vi "StartCAN.1.vi"(11 "CAN Interface":refnum<k21>="CAN1") -> (0 "error out":errorcluster, 1 "Tester Write Session out":refnum<k21>, 2 "Read Session out":refnum<k21>, 3 "DSC Write Session out":refnum<k21>)   [LabVIEW 2018]
uses:
  <vilib>/xnet/xnet.llb/XNET CAN Comm State.ctl
  <vilib>/xnet/xnet.llb/XNET Control Scope.ctl
  <vilib>/xnet/xnet.llb/XNET Frame CAN.ctl
  <vilib>/xnet/xnet.llb/XNET Frame Type CAN.ctl
  <vilib>/xnet/xnet.llb/XNET Create Session (Frame Input Queued).vi
  <vilib>/xnet/xnet.llb/XNET Create Session (Frame Output Single-point).vi
  <vilib>/xnet/xnet.llb/XNET Write (Frame CAN).vi
  <vilib>/xnet/xnet.llb/XNET Read (State CAN Comm).vi
  <vilib>/xnet/xnet.llb/XNET Wait (Interface Communicating).vi
  <resource>/objmgr/xnet.rc
panel:
  in  "error in (no error)":errorcluster
  out "TesterPresentSession":refnum<k21>
  out "CAN:I/O Mode":u32(ring) items=["CAN 2.0", "CAN FD", "CAN FD+BRS"]
  out "Protocol":u32(ring) items=["CAN", "FlexRay", "LIN"]
  out "CAN:Transceiver Capability":u32(ring) items=["HS"=0, "LS"=1, "XS"=3, "XS (HS/LS)"=4]
  out "Interface:CAN:Transceiver State":u32(ring) items=["Normal", "Sleep", "Single Wire Wakeup", "Single Wire High-Speed"]
  out "Interface:CAN:Transceiver State 2":u32(ring) items=["Normal", "Sleep", "Single Wire Wakeup", "Single Wire High-Speed"]
  out "Interface:CAN:Transceiver State 3":u32(ring) items=["Normal", "Sleep", "Single Wire Wakeup", "Single Wire High-Speed"]
  out "CAN:Termination Capability":u32(ring) items=["No", "Yes"]
  out "Array":T1[](array[typedef]) items=["Error Active", "Error Passive", "Bus Off", "Init"]
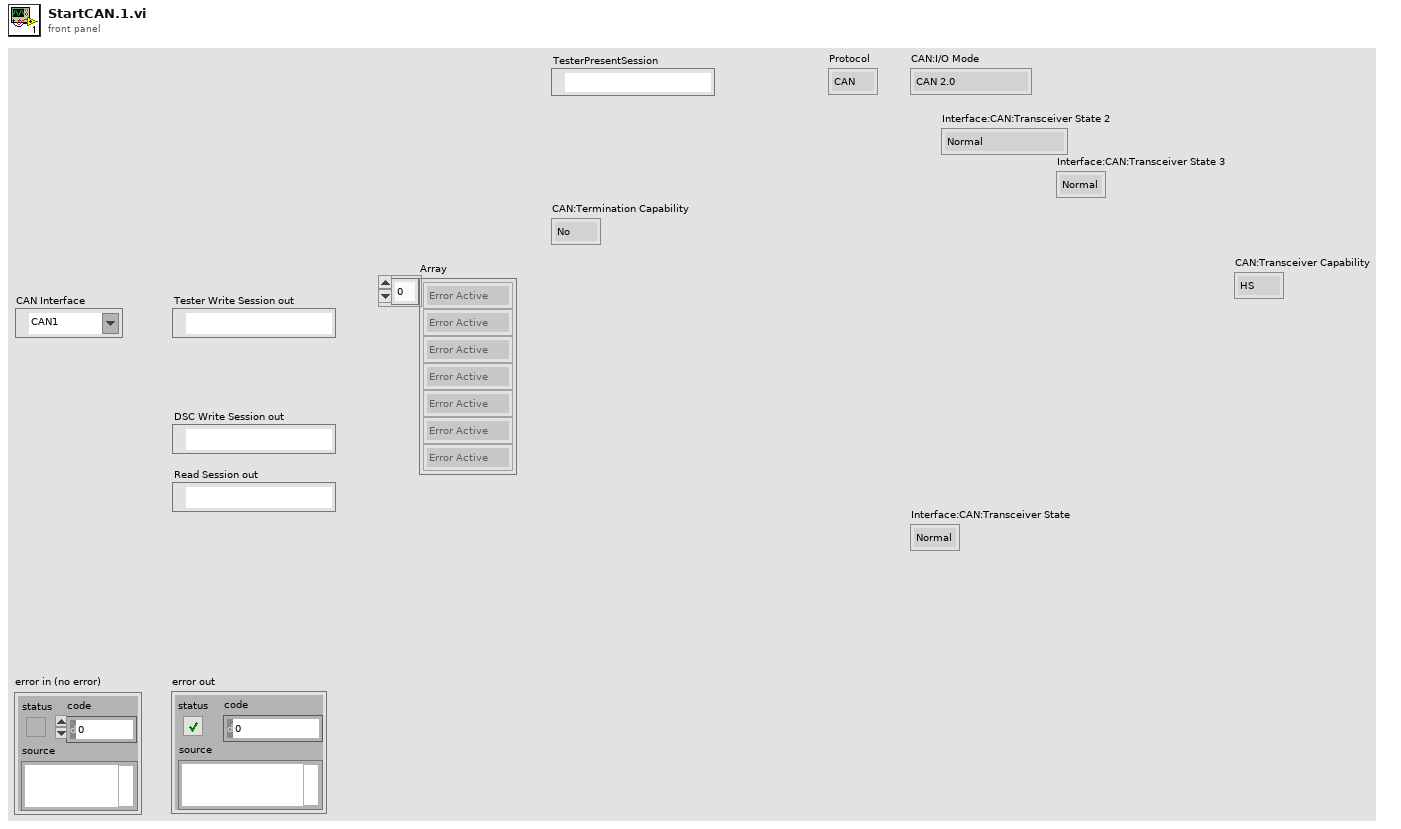
[diagram p1: front panel]
types:
  T1 = typedef "XNET CAN Comm State.ctl" = u8
  T2 = typedef "XNET Frame CAN.ctl" = cluster{"timestamp":timestamp, "payload":u8[], "identifier":u32, "type":T3, "extended?":bool, "echo?":bool}
  T3 = typedef "XNET Frame Type CAN.ctl" = u8
  T4 = typedef "XNET Control Scope.ctl" = u32
  T5 = cluster{"Comment":string, "Default Payload":u8[], "Identifier":u32, "Name (Short)":string, "Payload Length":u32, "PDU_Mapping":cluster{"PDU":string, "Start Bit":u32, "Update Bit":i32}[], "CAN:Extended Identifier?":bool, "CAN:Timing Type":u32, "CAN:Transmit Time":dbl, "CAN:I/O Mode":u32}
  T6 = typedef "XNET CAN Comm.ctl" = cluster{"fault code":i32, "fault?":bool, "communication state":T1, "last error":T7, "receive error counter":u8, "transmit error counter":u8, "transceiver error?":bool, "sleep?":bool}
  T7 = typedef "XNET CAN Last Err.ctl" = u8
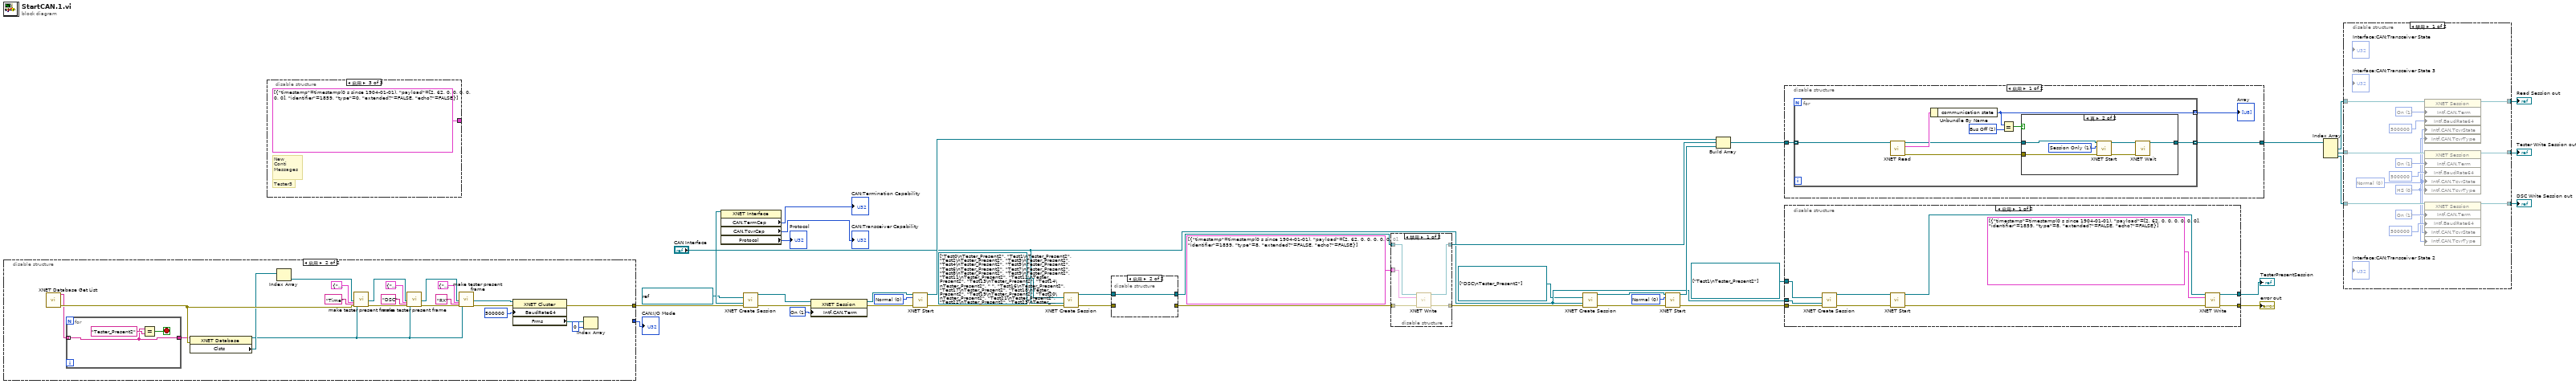
[diagram p0: block diagram]
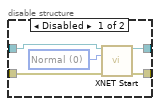
[diagram p3: hidden frame]
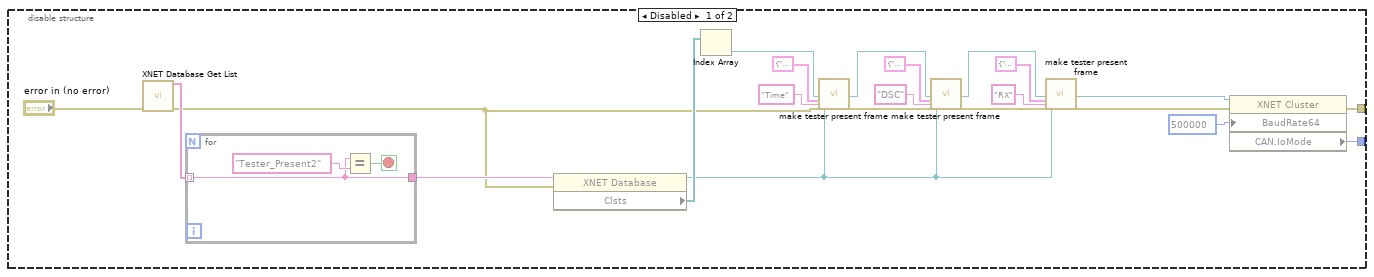
[diagram p4: hidden frame]
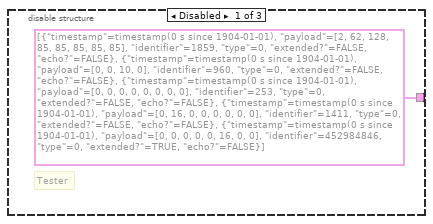
[diagram p9: hidden frame]
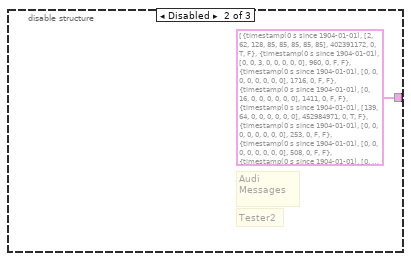
[diagram p10: hidden frame]
diagram:
  w11 = u32 1 items=["Off", "On"] ("Interface:CAN:Termination")
  w29 = T4 0 items=["Normal", "Session Only", "Interface Only", "Session Only Blocking"] ("scope (normal)")
  w30 = T4 0 items=["Normal", "Session Only", "Interface Only", "Session Only Blocking"] ("scope (normal)")
  n1 = disable-structure shown="启用" {
    disable-tunnel: [w60 w66] -> w40
    disable-tunnel: [w41 _] -> w15
    frame Disabled {
      n2 = call <vilib>:"XNET Database Get List.vi"("error in (no error)"="error in (no error)") -> ("array of alias"=w50:string[], "error out"=w46:errorcluster)  [unwired: 12 in, 1 out]
      n3 = for {
        tunnel: w50 -> [w63] mode=indexing
        tunnel: [w63] -> w49
        stop <- w64 stop-if-true
        n4 = Equal?(x=w63, y="Tester_Present2") -> (x = y?=w64:bool)
      }
      n5 = property class="XNET Database"(reference=w49, error in=w46) -> (reference out=w42:refnum<k21>, "Clsts"=w61:refnum<k21>[])  [unwired: 1 out]
      n6 = Index Array(array=w61) -> (element=w44:refnum<k21>)  [unwired: 1 in]
      n7 = call <userlib>:"make tester present frame.vi"("Cluster::"=w44, "New Frame Properties"=T5 {"Comment"="DSC", "Default Payload"=[0, 0, 0, 0, 0, 0, 0, 0], "Identifier"=1714, "Name (Short)"="Time", "Payload Length"=8, "PDU_Mapping"=[], "CAN:Extended Identifier?"=FALSE, "CAN:Timing Type"=0, "CAN:Transmit Time"=0.001, "CAN:I/O Mode"=0}, "frame name"="Time", "error in (no error)"=w46, "database in"=w42) -> ("target cluster out"=w43:refnum<k21>, "error out"=w45:errorcluster)  [unwired: 21 in]
      n8 = call <userlib>:"make tester present frame.vi"("Cluster::"=w43, "New Frame Properties"=T5 {"Comment"="DSC", "Default Payload"=[0, 0, 0, 0, 0, 0, 0, 0], "Identifier"=402391172, "Name (Short)"="DSC", "Payload Length"=8, "PDU_Mapping"=[], "CAN:Extended Identifier?"=TRUE, "CAN:Timing Type"=1, "CAN:Transmit Time"=0.001, "CAN:I/O Mode"=0}, "frame name"="DSC", "error in (no error)"=w45, "database in"=w42) -> ("target cluster out"=w59:refnum<k21>, "error out"=w58:errorcluster)  [unwired: 21 in]
      n9 = call <userlib>:"make tester present frame.vi"("Cluster::"=w59, "New Frame Properties"=T5 {"Comment"="RX", "Default Payload"=[0, 127, 0, 0, 0, 0, 0, 0], "Identifier"=402522244, "Name (Short)"="RX", "Payload Length"=8, "PDU_Mapping"=[], "CAN:Extended Identifier?"=TRUE, "CAN:Timing Type"=1, "CAN:Transmit Time"=0.001, "CAN:I/O Mode"=0}, "frame name"="RX", "error in (no error)"=w58, "database in"=w42) -> ("target cluster out"=w52:refnum<k21>, "error out"=w51:errorcluster)  [unwired: 21 in]
      n10 = property class="XNET Cluster"(reference=w52, error in=w51, "BaudRate64"=u64 500000 ("64bit Baud Rate")) -> (error out=w60:errorcluster, "CAN.IoMode"=w41:u32)  [unwired: 1 out]
    }
    frame Enabled {
      n11 = call <vilib>:"XNET Database Get List.vi"() -> ("array of alias"=w84:string[], "error out"=w85:errorcluster)  [unwired: 13 in, 1 out]
      n12 = for {
        tunnel: w84 -> [w88] mode=indexing
        tunnel: [w88] -> w71
        stop <- w89 stop-if-true
        n13 = Equal?(x=w88, y="Tester_Present2") -> (x = y?=w89:bool)
      }
      n14 = property class="XNET Database"(reference=w71, error in=w85) -> (reference out=w68:refnum<k21>, "Clsts"=w72:refnum<k21>[])  [unwired: 1 out]
      n15 = Index Array(array=w72) -> (element=w87:refnum<k21>)  [unwired: 1 in]
      n16 = call <userlib>:"make tester present frame.vi"("Cluster::"=w87, "New Frame Properties"=T5 {"Comment"="Time", "Default Payload"=[0, 0, 0, 0, 0, 0, 0, 0], "Identifier"=1859, "Name (Short)"="Time", "Payload Length"=8, "PDU_Mapping"=[], "CAN:Extended Identifier?"=FALSE, "CAN:Timing Type"=0, "CAN:Transmit Time"=0.1, "CAN:I/O Mode"=0}, "frame name"="Time", "error in (no error)"=w85, "database in"=w68) -> ("target cluster out"=w67:refnum<k21>, "error out"=w86:errorcluster)  [unwired: 21 in]
      n17 = call <userlib>:"make tester present frame.vi"("Cluster::"=w67, "New Frame Properties"=T5 {"Comment"="DSC", "Default Payload"=[0, 0, 0, 16, 1, 0, 0, 0], "Identifier"=1859, "Name (Short)"="DSC", "Payload Length"=8, "PDU_Mapping"=[], "CAN:Extended Identifier?"=FALSE, "CAN:Timing Type"=1, "CAN:Transmit Time"=0.001, "CAN:I/O Mode"=0}, "frame name"="DSC", "error in (no error)"=w86, "database in"=w68) -> ("target cluster out"=w80:refnum<k21>, "error out"=w81:errorcluster)  [unwired: 21 in]
      n18 = call <userlib>:"make tester present frame.vi"("Cluster::"=w80, "New Frame Properties"=T5 {"Comment"="RX", "Default Payload"=[0, 127, 0, 0, 0, 0, 0, 0], "Identifier"=1867, "Name (Short)"="RX", "Payload Length"=8, "PDU_Mapping"=[], "CAN:Extended Identifier?"=FALSE, "CAN:Timing Type"=1, "CAN:Transmit Time"=0.001, "CAN:I/O Mode"=0}, "frame name"="RX", "error in (no error)"=w81, "database in"=w68) -> ("target cluster out"=w82:refnum<k21>, "error out"=w83:errorcluster)  [unwired: 21 in]
      n19 = property class="XNET Cluster"(reference=w82, error in=w83, "BaudRate64"=u64 500000 ("64bit Baud Rate")) -> (error out=w66:errorcluster, "Frms"=w70:refnum<k21>[])  [unwired: 1 out]
      n20 = Index Array(array=w70, index=0 ("索引")) -> ()  [unwired: 1 out]
    }
  }
  "CAN:I/O Mode" <- w15
  n21 = disable-structure shown="启用" {
    disable-tunnel: [T2[] [{"timestamp"=timestamp(0 s since 1904-01-01), "payload"=[2, 62, 128, 85, 85, 85, 85, 85], "identifier"=1859, "type"=0, "extended?"=FALSE, "echo?"=FALSE}, {"timestamp"=timestamp(0 s since 1904-01-01), "payload"=[0, 0, 10, 0], "identifier"=960, "type"=0, "extended?"=FALSE, "echo?"=FALSE}, {"timestamp"=timestamp(0 s since 1904-01-01), "payload"=[0, 0, 0, 0, 0, 0, 0, 0], "identifier"=253, "type"=0, "extended?"=FALSE, "echo?"=FALSE}, {"timestamp"=timestamp(0 s since 1904-01-01), "payload"=[0, 16, 0, 0, 0, 0, 0, 0], "identifier"=1411, "type"=0, "extended?"=FALSE, "echo?"=FALSE}, {"timestamp"=timestamp(0 s since 1904-01-01), "payload"=[0, 0, 0, 0, 0, 16, 0, 0], "identifier"=452984846, "type"=0, "extended?"=TRUE, "echo?"=FALSE}] ("data") T2[] [{"timestamp"=timestamp(0 s since 1904-01-01), "payload"=[2, 62, 128, 85, 85, 85, 85, 85], "identifier"=402391172, "type"=0, "extended?"=TRUE, "echo?"=FALSE}, {"timestamp"=timestamp(0 s since 1904-01-01), "payload"=[0, 0, 3, 0, 0, 0, 0, 0], "identifier"=960, "type"=0, "extended?"=FALSE, "echo?"=FALSE}, {"timestamp"=timestamp(0 s since 1904-01-01), "payload"=[0, 0, 0, 0, 0, 0, 0, 0], "identifier"=1716, "type"=0, "extended?"=FALSE, "echo?"=FALSE}, {"timestamp"=timestamp(0 s since 1904-01-01), "payload"=[0, 16, 0, 0, 0, 0, 0, 0], "identifier"=1411, "type"=0, "extended?"=FALSE, "echo?"=FALSE}, {"timestamp"=timestamp(0 s since 1904-01-01), "payload"=[139, 64, 0, 0, 0, 0, 0, 0], "identifier"=452984971, "type"=0, "extended?"=TRUE, "echo?"=FALSE}, {"timestamp"=timestamp(0 s since 1904-01-01), "payload"=[0, 0, 0, 0, 0, 0, 0, 0], "identifier"=253, "type"=0, "extended?"=FALSE, "echo?"=FALSE}, {"timestamp"=timestamp(0 s since 1904-01-01), "payload"=[0, 0, 0, 0, 0, 0, 0, 0], "identifier"=508, "type"=0, "extended?"=FALSE, "echo?"=FALSE}, {"timestamp"=timestamp(0 s since 1904-01-01), "payload"=[0, 0, 0, 0, 150, 0, 0, 0], "identifier"=1646, "type"=0, "extended?"=FALSE, "echo?"=FALSE}, {"timestamp"=timestamp(0 s since 1904-01-01), "payload"=[0, 0, 0, 0, 0, 0, 0, 150], "identifier"=1719, "type"=0, "extended?"=FALSE, "echo?"=FALSE}, {"timestamp"=timestamp(0 s since 1904-01-01), "payload"=[0, 0, 4, 0, 0, 0, 0, 0], "identifier"=958, "type"=0, "extended?"=FALSE, "echo?"=FALSE}, {"timestamp"=timestamp(0 s since 1904-01-01), "payload"=[0, 0, 0, 0, 0, 0, 0, 0], "identifier"=1635, "type"=0, "extended?"=FALSE, "echo?"=FALSE}, {"timestamp"=timestamp(0 s since 1904-01-01), "payload"=[0, 0, 0, 0, 0, 0, 0, 0], "identifier"=319, "type"=0, "extended?"=FALSE, "echo?"=FALSE}, {"timestamp"=timestamp(0 s since 1904-01-01), "payload"=[0, 0, 0, 0, 0, 0, 0, 0], "identifier"=1616, "type"=0, "extended?"=FALSE, "echo?"=FALSE}, {"timestamp"=timestamp(0 s since 1904-01-01), "payload"=[0, 12, 0, 0, 0, 0, 0, 0], "identifier"=1413, "type"=0, "extended?"=FALSE, "echo?"=FALSE}, {"timestamp"=timestamp(0 s since 1904-01-01), "payload"=[0, 0, 0, 0, 0, 0, 0, 0], "identifier"=1462, "type"=0, "extended?"=FALSE, "echo?"=FALSE}, {"timestamp"=timestamp(0 s since 1904-01-01), "payload"=[16, 64, 0, 0, 0, 16, 0, 0], "identifier"=452984848, "type"=0, "extended?"=TRUE, "echo?"=FALSE}, {"timestamp"=timestamp(0 s since 1904-01-01), "payload"=[0, 0, 0, 0, 0, 0, 0, 0], "identifier"=976, "type"=0, "extended?"=FALSE, "echo?"=FALSE}, {"timestamp"=timestamp(0 s since 1904-01-01), "payload"=[0, 0, 0, 0, 0, 0, 0, 0], "identifier"=974, "type"=0, "extended?"=FALSE, "echo?"=FALSE}, {"timestamp"=timestamp(0 s since 1904-01-01), "payload"=[74, 64, 0, 0, 0, 0, 0, 0], "identifier"=452984906, "type"=0, "extended?"=TRUE, "echo?"=FALSE}, {"timestamp"=timestamp(0 s since 1904-01-01), "payload"=[0, 0, 0, 0, 0, 0, 0, 0], "identifier"=977, "type"=0, "extended?"=FALSE, "echo?"=FALSE}, {"timestamp"=timestamp(0 s since 1904-01-01), "payload"=[0, 0, 0, 0, 0, 0, 0, 0], "identifier"=975, "type"=0, "extended?"=FALSE, "echo?"=FALSE}, {"timestamp"=timestamp(0 s since 1904-01-01), "payload"=[75, 64, 0, 0, 0, 0, 0, 0], "identifier"=452984907, "type"=0, "extended?"=TRUE, "echo?"=FALSE}] ("Array 3") T2[] [{"timestamp"=timestamp(0 s since 1904-01-01), "payload"=[2, 62, 0, 0, 0, 0, 0, 0], "identifier"=1859, "type"=0, "extended?"=FALSE, "echo?"=FALSE}] ("data")] -> _
    frame Disabled {
      # "Tester"
    }
    frame Disabled {
      # "Tester2"
      # "Audi\nMessages"
    }
    frame Enabled {
      # "Tester3"
      # "New\nConti\nMessages"
    }
  }
  n22 = property class="XNET Interface"(reference="CAN Interface") -> ("CAN.TermCap"=→"CAN:Termination Capability":u32, "CAN.TcvrCap"=→"CAN:Transceiver Capability":u32, "Protocol"=→"Protocol":u32)  [unwired: 1 in, 2 out]
  n23 = call-poly <vilib>:"XNET Create Session.vi"("frame"=refnum<k21> "RX\nTester_Present2" ("XNET Frame"), "interface"="CAN Interface", "error in (no error)"=w40) -> ("session out"=w14:refnum<k21>, "error out"=w12:errorcluster)  [unwired: 11 in]
  n24 = property class="XNET Session"(reference=w14, error in=w12, "Intf.CAN.Term"=w11) -> (reference out=w13:refnum<k21>, error out=w10:errorcluster)
  n25 = call <vilib>:"XNET Start.vi"("session in"=w13, "scope (normal)"=w30, "error in (no error)"=w10) -> ("session out"=w37:refnum<k21>, "error out"=w32:errorcluster)  [unwired: 11 in]
  n26 = call-poly <vilib>:"XNET Create Session.vi"("frame list"=refnum<k21>[] ["Test0\nTester_Present2", "Test1\nTester_Present2", "Test2\nTester_Present2", "Test3\nTester_Present2", "Test4\nTester_Present2", "Test5\nTester_Present2", "Test6\nTester_Present2", "Test7\nTester_Present2", "Test8\nTester_Present2", "Test9\nTester_Present2", "Test11\nTester_Present2", "Test12\nTester_Present2", "Test13\nTester_Present2", "Test14\nTester_Present2", " ", "Test16\nTester_Present2", "Test17\nTester_Present2", "Test18\nTester_Present2", "Test19\nTester_Present2", "Test20\nTester_Present2", "Test21\nTester_Present2", "Test22\nTester_Present2", "Test23\nTester_Present2", "Test24\nTester_Present2", "Test25\nTester_Present2", "Test26\nTester_Present2", "Test27\nTester_Present2"] ("Frames"), "interface"="CAN Interface", "error in (no error)"=w32) -> ("session out"=w27:refnum<k21>, "error out"=w28:errorcluster)  [unwired: 11 in]
  n27 = disable-structure shown="启用" {
    disable-tunnel: [w98 w99] -> w39
    disable-tunnel: [w97 _] -> w38
    disable-tunnel: w28 -> [w95 _]
    disable-tunnel: w27 -> [w94 w99]
    frame Disabled {
      w96 = T4 0 items=["Normal", "Session Only", "Interface Only", "Session Only Blocking"] ("scope (normal)")
      n28 = call <vilib>:"XNET Start.vi"("session in"=w94, "scope (normal)"=w96, "error in (no error)"=w95) -> ("session out"=w98:refnum<k21>, "error out"=w97:errorcluster)  [unwired: 11 in]
    }
    frame Enabled {
    }
  }
  n29 = disable-structure shown="禁用" {
    disable-tunnel: w39 -> [w104 w105]
    disable-tunnel: w38 -> [w103 w106]
    disable-tunnel: [w102 w105] -> w36
    disable-tunnel: [w101 w106] -> w31
    disable-tunnel: T2[] [{"timestamp"=timestamp(0 s since 1904-01-01), "payload"=[2, 62, 0, 0, 0, 0, 0, 0], "identifier"=1859, "type"=8, "extended?"=FALSE, "echo?"=FALSE}] ("data") -> [w100 _]
    frame Disabled {
      n30 = call-poly <vilib>:"XNET Write.vi"("session in"=w104, "data"=w100, "error in (no error)"=w103) -> ("session out"=w102:refnum<k21>, "error out"=w101:errorcluster)  [unwired: 11 in]
    }
    frame Enabled {
    }
  }
  n31 = call-poly <vilib>:"XNET Create Session.vi"("frame list"=refnum<k21>[] ["DSC\nTester_Present2"] ("Frames"), "interface"="CAN Interface", "error in (no error)"=w31) -> ("session out"=w26:refnum<k21>, "error out"=w25:errorcluster)  [unwired: 11 in]
  n32 = call <vilib>:"XNET Start.vi"("session in"=w26, "scope (normal)"=w29, "error in (no error)"=w25) -> ("session out"=w35:refnum<k21>, "error out"=w6:errorcluster)  [unwired: 11 in]
  n33 = Build Array(w37, w36, w35) -> (w34:refnum<k21>[])
  n34 = disable-structure shown="启用" {
    disable-tunnel: w34 -> [w109 w125]
    disable-tunnel: [w107 w125] -> w33
    frame Enabled {
      n35 = for {
        tunnel: w109 -> [w116] mode=indexing
        tunnel: [w111] -> w108 mode=indexing
        tunnel: [w110] -> w107 mode=indexing
        w115 = T1 2 items=["Error Active", "Error Passive", "Bus Off", "Init"] ("y")
        n36 = call-poly <vilib>:"XNET Read.vi"("session in"=w116) -> ("session out"=w113:refnum<k21>, "CAN comm"=w117:T6, "error out"=w112:errorcluster)  [unwired: 12 in]
        n37 = Unbundle By Name(w117) -> ("communication state"=w111:T1)
        n38 = Equal?(x=w111, y=w115) -> (x = y?=w114:bool)
        n39 = case shown="真" w114 {
          tunnel: w113 -> [w118 w124]
          tunnel: w112 -> [_ w122]
          tunnel: [w118 w119] -> w110
          frame False {
          }
          frame True {
            w120 = T4 1 items=["Normal", "Session Only", "Interface Only", "Session Only Blocking"] ("scope (normal)")
            n40 = call <vilib>:"XNET Start.vi"("session in"=w124, "scope (normal)"=w120, "error in (no error)"=w122) -> ("session out"=w123:refnum<k21>, "error out"=w121:errorcluster)  [unwired: 11 in]
            n41 = call-poly <vilib>:"XNET Wait.vi"("session in"=w123, "error in (no error)"=w121) -> ("session out"=w119:refnum<k21>)  [unwired: 12 in, 1 out]
          }
        }
      }
      "Array" <- w108
    }
    frame Disabled {
    }
  }
  n42 = disable-structure shown="启用" {
    disable-tunnel: "CAN Interface" -> [w135 _]
    disable-tunnel: [w127 _] -> w8
    disable-tunnel: [w128 _] -> w7
    disable-tunnel: refnum<k21>[] ["Test1\nTester_Present2"] ("Frames") -> [w134 _]
    disable-tunnel: w6 -> [w131 _]
    frame Enabled {
      n43 = call-poly <vilib>:"XNET Create Session.vi"("frame list"=w134, "interface"=w135, "error in (no error)"=w131) -> ("session out"=w133:refnum<k21>, "error out"=w132:errorcluster)  [unwired: 11 in]
      n44 = call <vilib>:"XNET Start.vi"("session in"=w133, "error in (no error)"=w132) -> ("session out"=w130:refnum<k21>, "error out"=w129:errorcluster)  [unwired: 12 in]
      n45 = call-poly <vilib>:"XNET Write.vi"("session in"=w130, "data"=T2[] [{"timestamp"=timestamp(0 s since 1904-01-01), "payload"=[2, 62, 0, 0, 0, 0, 0, 0], "identifier"=1859, "type"=8, "extended?"=FALSE, "echo?"=FALSE}], "error in (no error)"=w129) -> ("session out"=w127:refnum<k21>, "error out"=w128:errorcluster)  [unwired: 11 in]
    }
    frame Disabled {
    }
  }
  "error out" <- w7
  "TesterPresentSession" <- w8
  n46 = Index Array(array=w33) -> (element #1=w23:refnum<k21>, element #2=w21:refnum<k21>, element #3=w19:refnum<k21>)  [unwired: 3 in]
  n47 = disable-structure shown="禁用" {
    disable-tunnel: w23 -> [w148 w152]
    disable-tunnel: [w147 w152] -> w22
    disable-tunnel: w21 -> [w144 w151]
    disable-tunnel: [w143 w151] -> w20
    disable-tunnel: w19 -> [w142 w150]
    disable-tunnel: [w141 w150] -> w18
    frame Disabled {
      w136 = u32 0 items=["HS", "LS", "SW", "Ext", "Disc"] ("Interface:CAN:Transceiver Type")
      w137 = u32 0 items=["Normal", "Sleep", "Single Wire Wakeup", "Single Wire High-Speed"] ("Interface:CAN:Transceiver State")
      w145 = u32 1 items=["Off", "On"] ("Interface:CAN:Termination")
      w146 = u32 1 items=["Off", "On"] ("Interface:CAN:Termination")
      w149 = u32 1 items=["Off", "On"] ("Interface:CAN:Termination")
      n48 = property class="XNET Session"(reference=w148, "Intf.CAN.Term"=w149, "Intf.BaudRate64"=u64 500000 ("Interface:64bit Baud Rate"), "Intf.CAN.TcvrState"=w137, "Intf.CAN.TcvrType"=w136) -> (reference out=w147:refnum<k21>)  [unwired: 1 in, 1 out]
      n49 = property class="XNET Session"(reference=w144, "Intf.CAN.Term"=w146, "Intf.BaudRate64"=u64 500000 ("Interface:64bit Baud Rate"), "Intf.CAN.TcvrState"=w137, "Intf.CAN.TcvrType"=w136) -> (reference out=w143:refnum<k21>)  [unwired: 1 in, 1 out]
      n50 = property class="XNET Session"(reference=w142, "Intf.CAN.Term"=w145, "Intf.BaudRate64"=u64 500000 ("Interface:64bit Baud Rate"), "Intf.CAN.TcvrState"=w137, "Intf.CAN.TcvrType"=w136) -> (reference out=w141:refnum<k21>)  [unwired: 1 in, 1 out]
    }
    frame Enabled {
    }
  }
  "Tester Write Session out" <- w20
  "Read Session out" <- w22
  "DSC Write Session out" <- w18
